vi "listen_tcp_data_conn.vi"(8 "error in":errorcluster, 9 "TCP output port":i32=6666, 10 "TCP input port":i32=6666) -> (0 "error out":errorcluster)   [LabVIEW 2014]
uses:
  ilemt_globals.vi
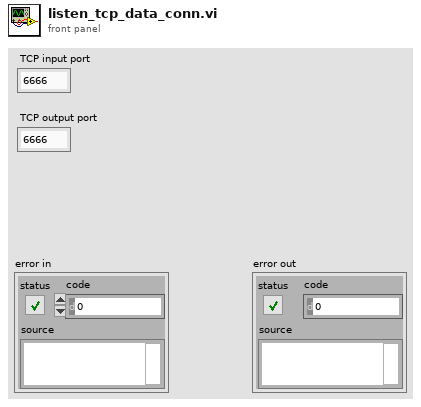
[diagram p1: front panel]
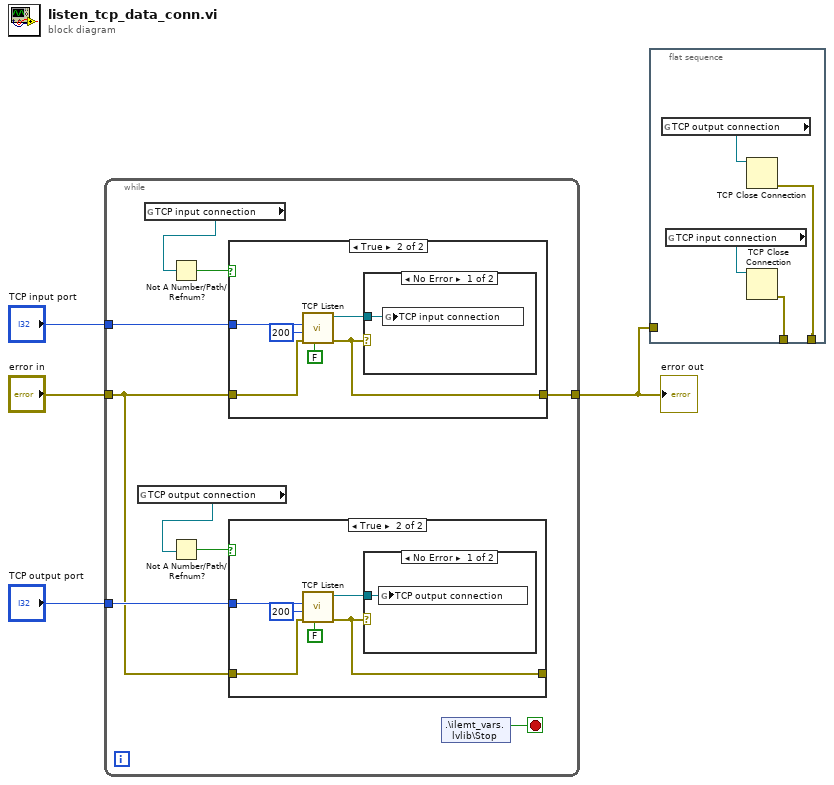
[diagram p0: block diagram]
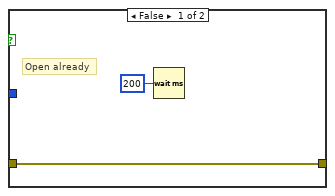
[diagram p2: hidden frame]
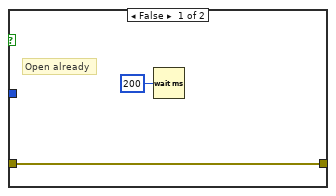
[diagram p4: hidden frame]
diagram:
  n1 = while {
    tunnel: "TCP input port" -> [w11]
    tunnel: "error in" -> [w6]
    tunnel: [w10] -> w2
    tunnel: "TCP output port" -> [w7]
    stop <- w9 stop-if-true
    n2 = global read "ilemt_globals.vi" "TCP output connection"() -> (w5:refnum<k5>)
    n3 = global read "ilemt_globals.vi" "TCP input connection"() -> (w13:refnum<k5>)
    n4 = Not A Number/Path/Refnum?(number/path/refnum=w13) -> (NaN/Path/Refnum?=w12:bool)
    n5 = Not A Number/Path/Refnum?(number/path/refnum=w5) -> (NaN/Path/Refnum?=w8:bool)
    n6 = case shown="True" w12 {
      tunnel: w11 -> [_ w30]
      tunnel: w6 -> [w24 w28]
      tunnel: [w24 w25] -> w10
      frame False {
        # "Open already"
        n7 = Wait (ms)(milliseconds to wait=u32 200) -> ()  [unwired: 1 out]
      }
      frame True {
        n8 = call <vilib>:"TCP Listen.vi"("resolve remote address (T)"=FALSE, "error in (no error)"=w28, "timeout ms (wait forever: -1)"=200, "port"=w30) -> ("error out"=w25:errorcluster, "connection ID"=w26:refnum<k5>)  [unwired: 3 in, 3 out]
        n9 = case shown="No Error" w25 {
          tunnel: w26 -> [w31 _]
          frame No Error {
            n10 = global write "ilemt_globals.vi" "TCP input connection"(w31) -> ()
          }
          frame Error {
          }
        }
      }
    }
    n11 = case shown="True" w8 {
      tunnel: w7 -> [_ w21]
      tunnel: w6 -> [w15 w19]
      tunnel: [w15 w16] -> _
      frame False {
        # "Open already"
        n12 = Wait (ms)(milliseconds to wait=u32 200) -> ()  [unwired: 1 out]
      }
      frame True {
        n13 = call <vilib>:"TCP Listen.vi"("resolve remote address (T)"=FALSE, "error in (no error)"=w19, "timeout ms (wait forever: -1)"=200, "port"=w21) -> ("error out"=w16:errorcluster, "connection ID"=w17:refnum<k5>)  [unwired: 3 in, 3 out]
        n14 = case shown="No Error" w16 {
          tunnel: w17 -> [w22 _]
          frame No Error {
            n15 = global write "ilemt_globals.vi" "TCP output connection"(w22) -> ()
          }
          frame Error {
          }
        }
      }
    }
    n16 = shared-variable ".\\ilemt_vars.lvlib\\Stop"() -> (w9:bool)  [unwired: 1 in, 1 out]
  }
  "error out" <- w2
  n17 = flat-sequence {
    tunnel: w2 -> [_]
    tunnel: [w34] -> _
    tunnel: [w32] -> _
    frame #0 {
      n18 = global read "ilemt_globals.vi" "TCP output connection"() -> (w33:refnum<k5>)
      n19 = global read "ilemt_globals.vi" "TCP input connection"() -> (w35:refnum<k5>)
      n20 = TCP Close Connection(connection ID=w33) -> (error out=w32:errorcluster)  [unwired: 1 in, 2 out]
      n21 = TCP Close Connection(connection ID=w35) -> (error out=w34:errorcluster)  [unwired: 1 in, 2 out]
    }
  }
